vi "DIFF_DRIVE_GET_MAX.vi"() -> (1 "Max Rotational Vel (Rad/Sec)":dbl, 3 "Max Wheel Vel (Meter/Sec)":dbl)   [LabVIEW 2023]
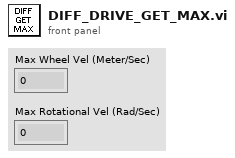
[diagram p1: front panel]
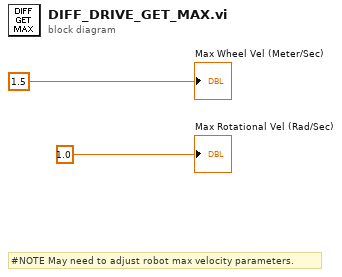
[diagram p0: block diagram]
diagram:
  # "#NOTE May need to adjust robot max velocity parameters."
  "Max Wheel Vel (Meter/Sec)" <- 1.5
  "Max Rotational Vel (Rad/Sec)" <- 1.0 ("Max Rotational Vel (Rad/Sec)")
